vi "Subvi probes DIO24-31 D7-0.vi"() -> ()   [LabVIEW 2017]
uses:
  <vilib>/rvi/eio/common/nirviEmuTemplateMethod_errors.vi
  <vilib>/eio/EIONode/EIONode.xnode
panel:
  in  "DIO31":bool
  in  "DIO30":bool
  in  "DI029":bool
  in  "DIO28":bool
  in  "DIO27":bool
  in  "DIO26":bool
  in  "DIO25":bool
  in  "DIO24":bool
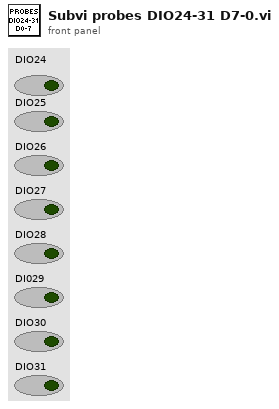
[diagram p1: front panel]
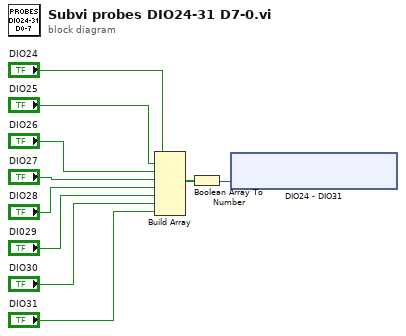
[diagram p0: block diagram]
diagram:
  n1 = Build Array("DIO24", "DIO25", "DIO26", "DIO27", "DIO28", "DI029", "DIO30", "DIO31") -> (w10:bool[])
  n2 = Boolean Array To Number(Boolean array=w10) -> (number=w9:u8)
  n3 = xnode "DIO24 - DIO31"("Connector0/DIOPORT3"=w9) -> ()  [unwired: 1 in, 1 out]
